vi "String decode.vi"(0 "INPUT String":string="##@22/06/29 17:39:36;0.8800000000000003;34.40;0.098;44.98465;4.4084957000000005;5701.223688000001;{0.001,-0.034,-0.003,0.005,-0.122,-0.194,-0.134,0.040,-0.042,-0.055,0.195,0.307,0.229,0.199,0.308,0.175,0.229,0.423,0.252,0.074,}") -> (14 "new data?":bool, 15 "data":T1)   [LabVIEW 2022 SP3, in "LS-H600-TCP Client.lvlib" / "LS-H600-TCP Client.lvclass"]
uses:
  LS-H600-TCP Client.lvclass
panel:
  # "数据时间\n仪器水深\n水温\n流速\n过水面积\n瞬时流量\n累积流量\n剖面流速"
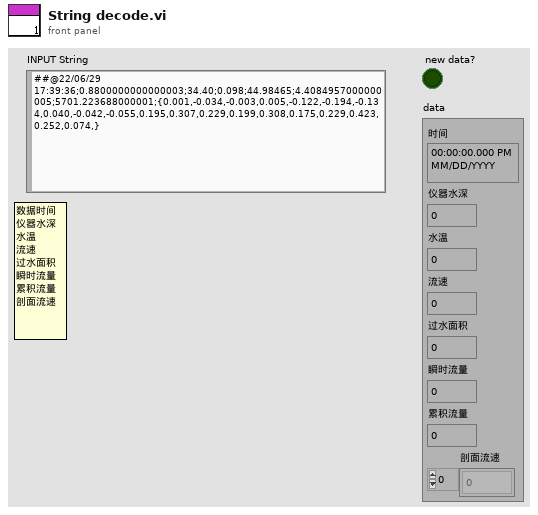
[diagram p1: front panel]
types:
  T1 = cluster{"时间":timestamp, "仪器水深":dbl, "水温":dbl, "流速":dbl, "过水面积":dbl, "瞬时流量":dbl, "累积流量":dbl, "剖面流速":dbl[]}
  T2 = cluster{"时间标识":timestamp, dbl, dbl, dbl, dbl, dbl, dbl, dbl[]}
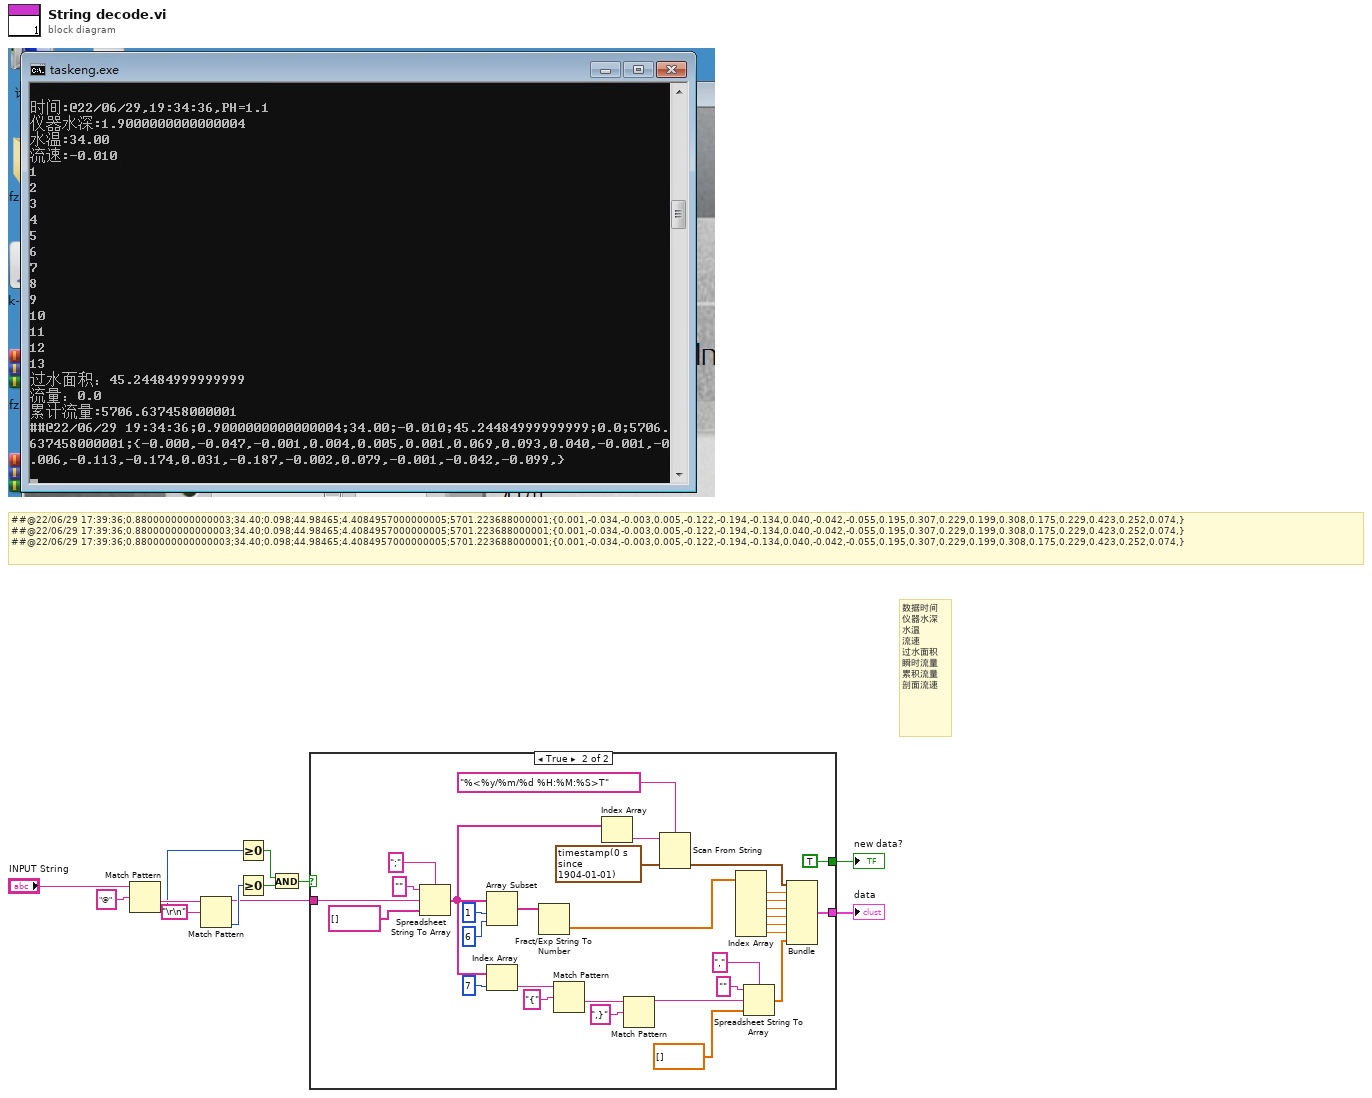
[diagram p0: block diagram]
diagram:
  # "数据时间\n仪器水深\n水温\n流速\n过水面积\n瞬时流量\n累积流量\n剖面流速"
  # "##@22/06/29 17:39:36;0.8800000000000003;34.40;0.098;44.98465;4.4084957000000005;5701.223688000001;{0.001,-0.034,-0.003,0.005,-0.122,-0.194,-0.134,0.040,-0.042,-0.055,0.195,0.307,0.229,0.199,0.308,0.175,0.229,0.423,0.252,0.074,}\n##@22/06/29 17:39:36;0.8800000000000003;34.40;0.098;44.98465;4.4084957000000005;5701.223688000001;{0.001,-0.034,-0.003,0.005,-0.122,-0.194,-0.134,0.040,-0.042,-0.055,0.195,0.307,0.229,0.199,0.308,0.175,0.229,0.423,0.252,0.074,}\n##@22/06/29 17:39:36;0.8800000000000003;34.40;0.098;44.98465;4.4084957000000005;5701.223688000001;{0.001,-0.034,-0.003,0.005,-0.122,-0.194,-0.134,0.040,-0.042,-0.055,0.195,0.307,0.229,0.199,0.308,0.175,0.229,0.423,0.252,0.074,}"
  n1 = Match Pattern(string="INPUT String", regular expression="@" ("正则表达式")) -> (after substring=w9:string, offset past match=w7:i32)  [unwired: 1 in, 2 out]
  n2 = Match Pattern(string=w9, regular expression="\r\n") -> (before substring=w2:string, offset past match=w6:i32)  [unwired: 1 in, 2 out]
  n3 = Greater Or Equal To 0?(x=w7) -> (x >= 0?=w4:bool)
  n4 = Greater Or Equal To 0?(x=w6) -> (x >= 0?=w5:bool)
  n5 = And(x=w4, y=w5) -> (x .and. y?=w3:bool)
  n6 = case shown="True" w3 {
    tunnel: [_ w16] -> w12
    tunnel: w2 -> [_ w14]
    tunnel: [_ TRUE] -> w1
    frame False {
    }
    frame True {
      n7 = Spreadsheet String To Array(delimiter (Tab)=";" ("分隔符(Tab)"), format string="" ("格式字符串"), spreadsheet string=w14, array type (2D Dbl)=string[] []) -> (array=w35:string[])
      n8 = Array Subset(array=w35, index=1 ("索引"), length=6 ("长度")) -> (w36:string[])
      n9 = Index Array(array=w35, index=7 ("索引")) -> (element=w33:string)
      n10 = Fract/Exp String To Number(string=w36) -> (number=w24:dbl[])  [unwired: 3 in, 1 out]
      n11 = Match Pattern(string=w33, regular expression="{" ("正则表达式")) -> (after substring=w28:string)  [unwired: 1 in, 3 out]
      n12 = Index Array(array=w35) -> (element=w15:string)  [unwired: 1 in]
      n13 = Match Pattern(string=w28, regular expression=",}" ("正则表达式")) -> (before substring=w26:string)  [unwired: 1 in, 3 out]
      n14 = Scan From String(format string="%<%y/%m/%d %H:%M:%S>T" ("格式字符串"), input string=w15, default 1=timestamp(0 s since 1904-01-01) ("时间标识")) -> (output 1=w25:timestamp)  [unwired: 2 in, 3 out]
      n15 = Index Array(array=w24) -> (element #1=w23:dbl, element #2=w22:dbl, element #3=w21:dbl, element #4=w20:dbl, element #5=w19:dbl, element #6=w18:dbl)  [unwired: 6 in]
      n16 = Spreadsheet String To Array(delimiter (Tab)="," ("分隔符(Tab)"), format string="" ("格式字符串"), spreadsheet string=w26, array type (2D Dbl)=dbl[] []) -> (array=w17:dbl[])
      n17 = Bundle("时间标识"=w25, w23, w22, w21, w20, w19, w18, w17) -> (w16:T2)  [unwired: 1 in]
    }
  }
  "data" <- w12
  "new data?" <- w1
